vi "Command_Turn_To_Heading_Simplevi.vi"(6 "Timeout":dbl=3.0, 8 "Speed":dbl=1.0, 9 "Heading":dbl=-20.0, 11 "Startup":bool) -> (0 "Right Wheel":dbl, 1 "Reinit":bool, 2 "Left Wheel":dbl, 3 "Completed":bool=TRUE)   [LabVIEW 2019]
uses:
  Subsystems/Sensing/Sensor_Values.vi
panel:
  in  "Turn_To_Heading_Acceptable_Error":dbl
  in  "Turn Gain":dbl=0.06
  # "Alpha .06"
  # "Beta .1"
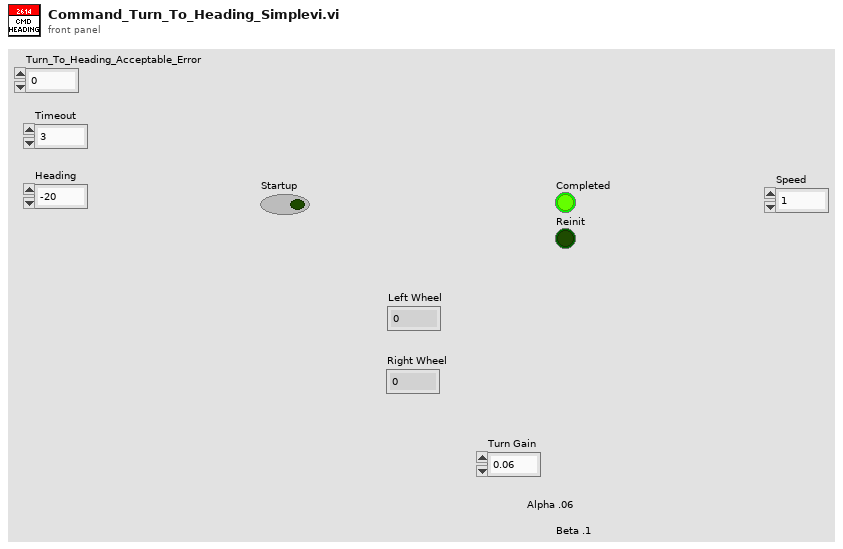
[diagram p1: front panel]
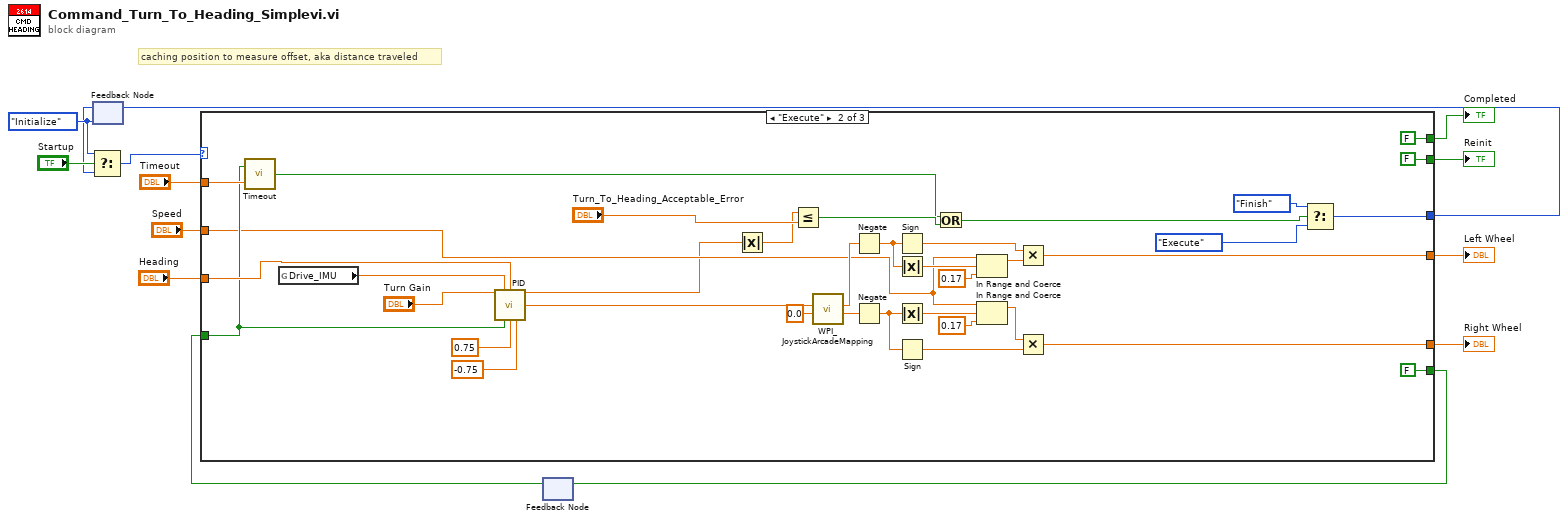
[diagram p0: block diagram]
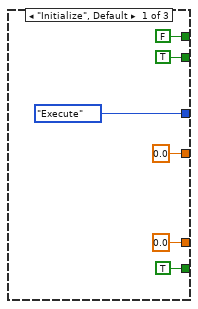
[diagram p2: hidden frame]
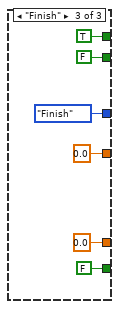
[diagram p3: hidden frame]
diagram:
  w12 = enum16{"Initialize", "Execute", "Finish"}."Initialize"
  # "caching position to measure offset, aka distance traveled"
  n1 = feedback #1(w12) -> (w8:enum16{"Initialize", "Execute", "Finish"})
  n2 = Select(t=w12, s="Startup", f=w8) -> (s? t:f=w13:enum16{"Initialize", "Execute", "Finish"})
  n3 = feedback #2() -> (w3:bool)  [unwired: 1 in]
  n4 = case shown="\"Execute\"" w13 {
    tunnel: [FALSE FALSE TRUE] -> w11
    tunnel: [TRUE FALSE FALSE] -> w10
    tunnel: [enum16{"Initialize", "Execute", "Finish"}."Execute" w53 enum16{"Initialize", "Execute", "Finish"}."Finish"] -> w9
    tunnel: [0.0 ("Left Wheel Velocity") w30 0.0] -> w7
    tunnel: [0.0 ("Right Wheel Velocity") w31 0.0] -> w6
    tunnel: "Heading" -> [_ w48 _]
    tunnel: [TRUE FALSE FALSE] -> w4
    tunnel: w3 -> [_ w32 _]
    tunnel: "Timeout" -> [_ w43 _]
    tunnel: "Speed" -> [_ w29 _]
    frame "Initialize", Default {
    }
    frame "Execute" {
      n5 = call "Timeout.vi"("Timeout"=w43, "Initialize"=w32) -> ("Timed Out?"=w22:bool)
      n6 = global read "Sensor_Values.vi" "Drive_IMU"() -> (w28:dbl)
      n7 = call "PID.vi"("Kp"="Turn Gain", "Process Variable"=w28, "Goal"=w48, "Reinit"=w32, "Max Ouput"=0.75, "Min Output"=-0.75) -> ("Current Error"=w25:dbl, "Command"=w47:dbl)  [unwired: 7 in, 1 out]
      n8 = Absolute Value(x=w25) -> (abs(x)=w24:dbl)
      n9 = Less Or Equal?(x=w24, y="Turn_To_Heading_Acceptable_Error") -> (x <= y?=w23:bool)
      n10 = call <vilib>:"WPI_JoystickArcadeMapping.vi"("Y axis value"=0.0, "X axis value"=w47) -> ("Right Motor Value"=w45:dbl, "Left Motor Value"=w46:dbl)  [unwired: 8 in]
      n11 = Negate(x=w46) -> (-x=w39:dbl)
      n12 = Negate(x=w45) -> (-x=w40:dbl)
      n13 = Sign(1:w39) -> (0:w38:dbl)
      n14 = Absolute Value(x=w39) -> (abs(x)=w42:dbl)
      n15 = Absolute Value(x=w40) -> (abs(x)=w41:dbl)
      n16 = Sign(1:w40) -> (0:w35:dbl)
      n17 = Or(x=w22, y=w23) -> (x .or. y?=w21:bool)
      n18 = In Range and Coerce(upper limit=w29, x=w42, lower limit=0.17) -> (coerced(x)=w37:dbl)  [unwired: 1 out]
      n19 = In Range and Coerce(upper limit=w29, x=w41, lower limit=0.17) -> (coerced(x)=w36:dbl)  [unwired: 1 out]
      n20 = Multiply(x=w38, y=w37) -> (x*y=w30:dbl)
      n21 = Multiply(x=w36, y=w35) -> (x*y=w31:dbl)
      n22 = Select(t=enum16{"Initialize", "Execute", "Finish"}."Finish", s=w21, f=enum16{"Initialize", "Execute", "Finish"}."Execute") -> (s? t:f=w53:enum16{"Initialize", "Execute", "Finish"})
    }
    frame "Finish" {
    }
  }
  "Completed" <- w11
  "Reinit" <- w10
  "Left Wheel" <- w7
  "Right Wheel" <- w6
  n23 = feedback-in #1(w9) -> ()
  n24 = feedback-in #2(w4) -> ()
